vi "Wait Until Connected.vi"(8 "error in (no error)":errorcluster, 10 "timeout in ms (-1)":i32=-1, 11 "input in":refnum<class "Input.lvclass">) -> (0 "error out":errorcluster, 2 "timeout":bool, 3 "input out":refnum<class "Input.lvclass">)   [LabVIEW 2015, in "Input.lvclass"]
uses:
  Input.lvclass
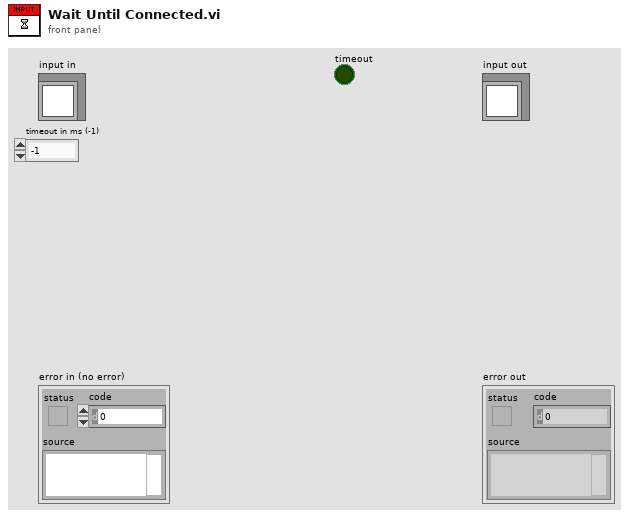
[diagram p1: front panel]
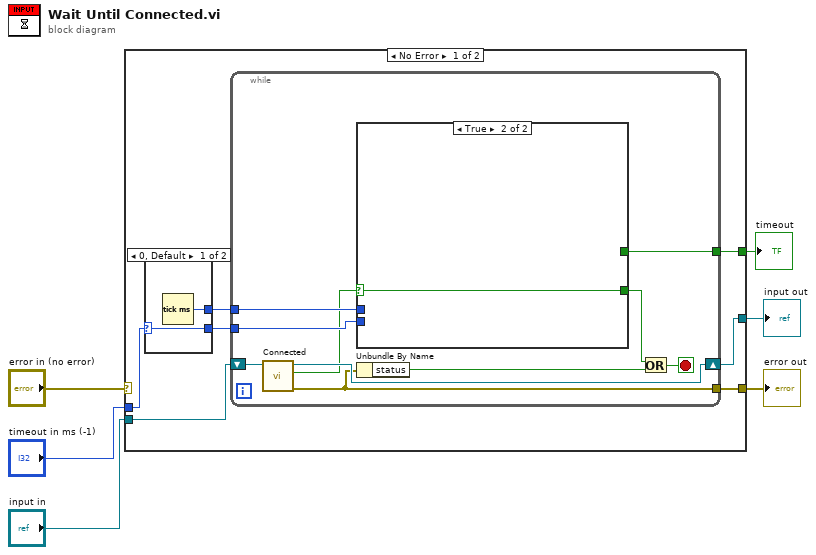
[diagram p0: block diagram]
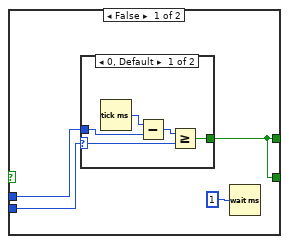
[diagram p3: hidden frame]
diagram:
  n1 = case shown="No Error" "error in (no error)" {
    selector: "error in (no error)" -> [_ w38]
    tunnel: [w8 w38] -> w5
    tunnel: [w9 w37] -> w3
    tunnel: "input in" -> [w13 w37]
    tunnel: "timeout in ms (-1)" -> [w12 _]
    tunnel: [w7 _] -> w1
    frame No Error {
      n2 = case shown="0, Default" w12 {
        selector: w12 -> [w15 w16]
        tunnel: [w15 w16] -> w11
        tunnel: [w14 _] -> w10
        frame 0, Default {
          n3 = Tick Count (ms)() -> (millisecond timer value=w14:u32)
        }
        frame -1 {
        }
      }
      n4 = while {
        tunnel: w11 -> [w25]
        tunnel: w10 -> [w24]
        shift-right: [w23] -> w9
        shift-left: w13 -> [w26]
        tunnel: [w18] -> w8
        tunnel: [w17] -> w7
        stop <- w19 stop-if-true
        n5 = call "Connected.vi"("input in"=w26) -> ("error out"=w18:errorcluster, "connected"=w22:bool, "input out"=w23:refnum<class "Input.lvclass">)  [unwired: 8 in]
        n6 = case shown="True" w22 {
          selector: w22 -> [_ w36]
          tunnel: w25 -> [w30 _]
          tunnel: w24 -> [w29 _]
          tunnel: [w27 w36] -> w21
          tunnel: [w27 _] -> w17
          frame False {
            n7 = case shown="0, Default" w30 {
              selector: w30 -> [w32 _]
              tunnel: w29 -> [w35 _]
              tunnel: [w31 _] -> w27
              frame 0, Default {
                n8 = Tick Count (ms)() -> (millisecond timer value=w34:u32)
                n9 = Subtract(x=w34, y=w35) -> (x-y=w33:u32)
                n10 = Greater Or Equal?(x=w33, y=w32) -> (x >= y?=w31:bool)
              }
              frame -1 {
              }
            }
            n11 = Wait (ms)(milliseconds to wait=u32 1) -> ()  [unwired: 1 out]
          }
          frame True {
          }
        }
        n12 = Unbundle By Name(w18) -> ("status"=w20:bool)
        n13 = Or(x=w21, y=w20) -> (x .or. y?=w19:bool)
      }
    }
    frame Error {
    }
  }
  "error out" <- w5
  "input out" <- w3
  "timeout" <- w1
